vi "update.assets.request.vi"(8 "error in":errorcluster, 11 "Assets":refnum<class "asset.lvclass">[](array[class])) -> (0 "error out":errorcluster, 3 "request":string)   [LabVIEW 2020, in "Run.lvclass"]
uses:
  Run.lvclass
  asset/asset.lvclass
  asset/asset.lvclass/asset.ctl
  asset/rid.get.vi
  846ed7e2-8c26-4a38-8561-4cc48212a6c5.vi
  <vilib>/JDP Science/JSONtext/Variant to JSON Text.vi
  <vilib>/JDP Science/JSONtext/support/Format JSON Object.vi
  <vilib>/JDP Science/JSONtext/LVClass Serializer/JSONtext LVClass Serializer.lvclass
  <vilib>/JDP Science/JSONtext/JSONtext.lvlib
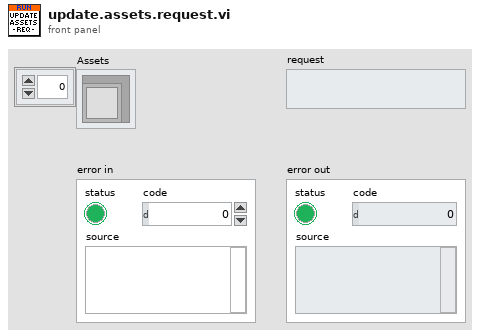
[diagram p1: front panel]
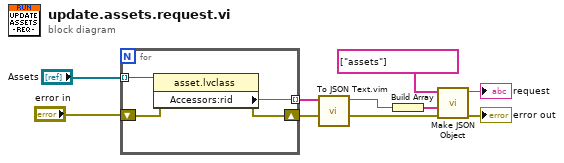
[diagram p0: block diagram]
diagram:
  n1 = for {
    tunnel: "Assets" -> [w14] mode=indexing
    tunnel: [w13] -> w9 mode=indexing
    shift-right: [w12] -> w3
    shift-left: "error in" -> [w11]
    n2 = property class="asset.lvclass"(reference=w14, error in=w11) -> (error out=w12:errorcluster, "Accessors:rid"=w13:string)  [unwired: 1 out]
  }
  n3 = call "To JSON Text.vim"("error in (no error)"=w3, "Anything"=w9) -> ("error out"=w4:errorcluster, "<JSON>"=w6:string)  [unwired: 8 in]
  n4 = Build Array(w6) -> (w7:string[])
  n5 = call <vilib>:"Make JSON Object.vi"("error in (no error)"=w4, "JSON Items"=w7, "Item Names"=string[] ["assets"]) -> ("error out"=→"error out":errorcluster, "<JSON>"=→"request":string)  [unwired: 7 in]
